vi "Assert Test In Loop.vi"(8 "error in (no error)":errorcluster) -> (0 "error out":errorcluster)   [LabVIEW 2009, in "test-lvlib.lvlib"]
uses:
  test-lvlib.lvlib
  classes/Assert/Assert.lvclass
  classes/Test/Test.lvclass
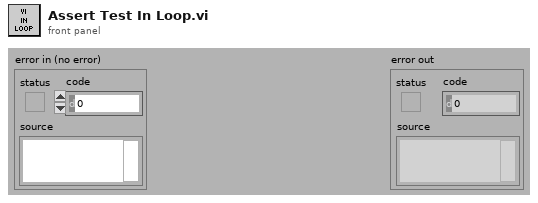
[diagram p1: front panel]
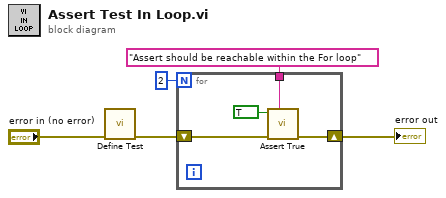
[diagram p0: block diagram]
diagram:
  n1 = call "Define Test.vi"("error in (no error)"="error in (no error)") -> ("error out"=w3:errorcluster)  [unwired: 10 in]
  n2 = for {
    N: 2 -> [_]
    tunnel: "Assert should be reachable within the For loop" ("Label") -> [w8]
    shift-right: [w6] -> w1
    shift-left: w3 -> [w7]
    n3 = call "Assert True.vi"("Label"=w8, "error in (no error)"=w7, "True?"=TRUE) -> ("error out"=w6:errorcluster)  [unwired: 8 in]
  }
  "error out" <- w1
